vi "Example.vi"() -> ()   [LabVIEW 2014, in "Nephelometer.lvclass"]
uses:
  Nephelometer.lvclass
  Reusable/Session APIs/File Access/Config Data/Config Session.ctl
  Reusable/Session APIs/File Access/Config Data/Config Data.lvclass
  Configurable Device/Configurable Device.lvclass/Configurable Device.ctl
  Reusable/Session APIs/Serial/Serial Session.lvclass
  Nephelometer.lvclass/Nephelometer.ctl
  Configurable Device/Write Handle.vi
  <userlib>/_Session Fwk/Session - Root.lvclass
panel:
  out "error out 6":errorcluster
  in  "Fan Power":bool
  in  "Lamp Power":bool
  in  "position":enum16{"Total", "Back"}(ring)
  in  "Power":bool=TRUE
  out "Aux Data":T1
  out "Data Record":T2
  in  "Zero":bool
  out "Autozero Mode":i32
  out "error out 5":errorcluster
  out "current time":timestamp
  out "error out 4":errorcluster
  out "error out 3":errorcluster
  in  "Valve":bool
  in  "Blower":u8(slide) scale=0.0..255.0
  out "error out":errorcluster
  out "Vlamp":cluster{"Voltage":dbl, "Amperage":dbl}
  out "Tsample":dbl
  out "Tinlet":dbl
  out "RH":dbl
  out "Pressure":dbl
  out "error out 2":errorcluster
  out "RD":string
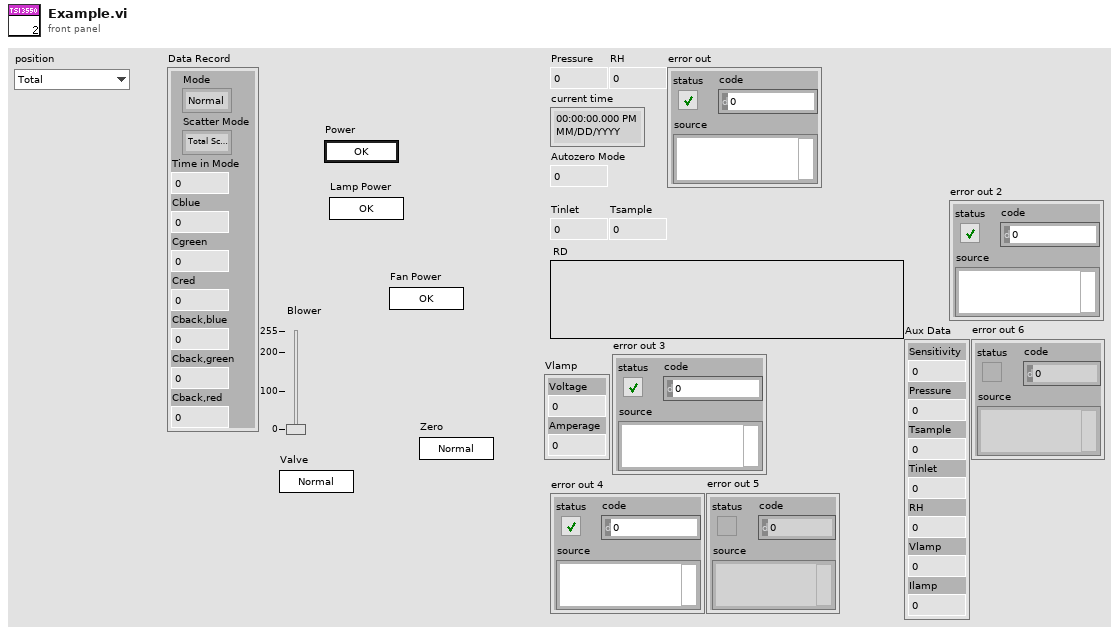
[diagram p1: front panel]
types:
  T1 = cluster{"Sensitivity":dbl, "Pressure":dbl, "Tsample":dbl, "Tinlet":dbl, "RH":dbl, "Vlamp":dbl, "Ilamp":dbl}
  T2 = cluster{"Mode":enum16{"Normal", "Zero", "Blank"}, "Scatter Mode":enum16{"Total Scatter", "Back Scatter"}, "Time in Mode":dbl, "Cblue":i32, "Cgreen":dbl, "Cred":dbl, "Cback,blue":dbl, "Cback,green":dbl, "Cback,red":dbl}
  T3 = typedef "Config Data.lvclass/Config Session.ctl" = refnum<data-value>
  T4 = typedef "Session - Root.lvclass/Session Handle.ctl" = refnum<data-value>
  T5 = cluster{"Mode":enum16{"Normal", "Zero", "Blank"}, "Scatter Mode":enum16{"Total Scatter", "Back Scatter"}, "Time in Mode":i32, "Cblue":dbl, "Cgreen":dbl, "Cred":dbl, "Cback,blue":dbl, "Cback,green":dbl, "Cback,red":dbl}
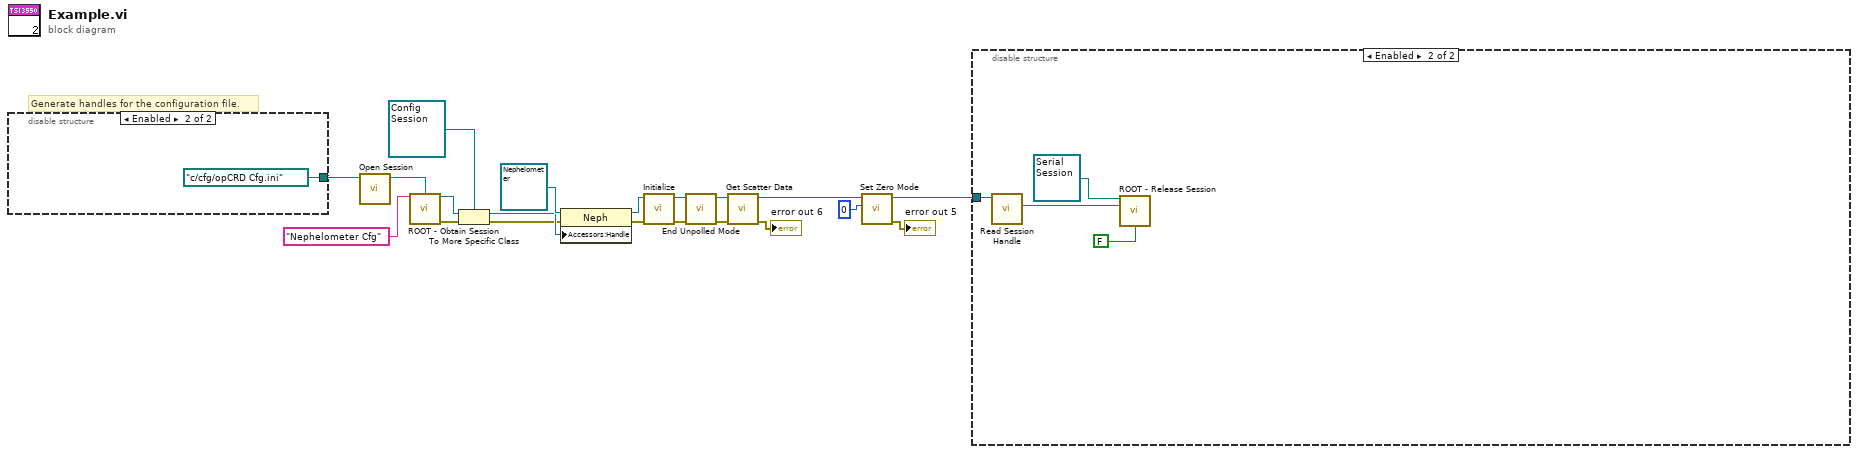
[diagram p0: block diagram]
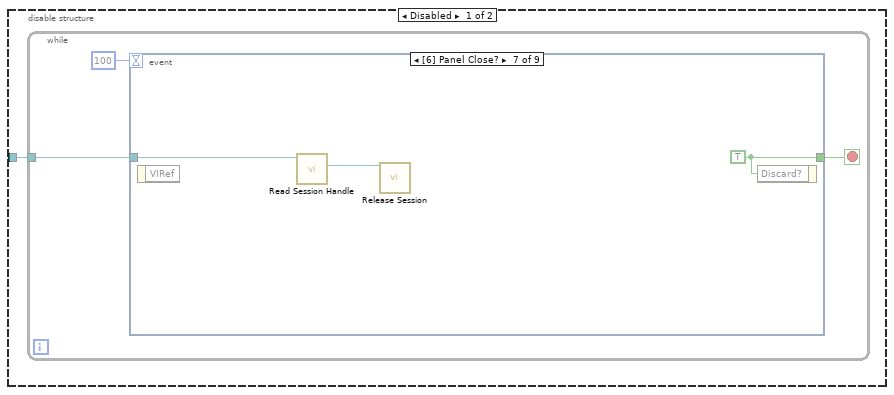
[diagram p2: hidden frame]
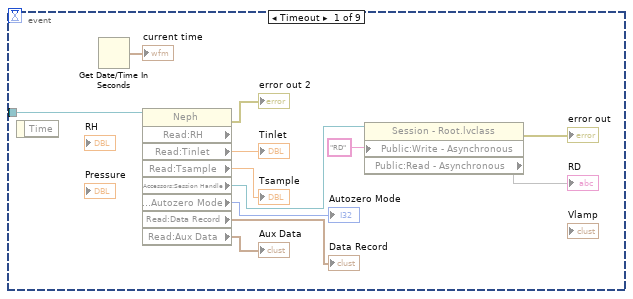
[diagram p3: hidden frame]
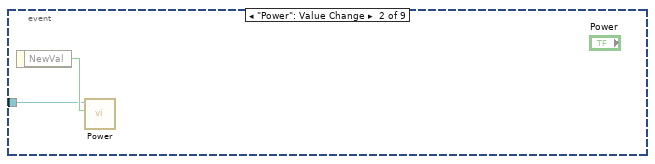
[diagram p4: hidden frame]
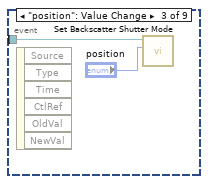
[diagram p5: hidden frame]
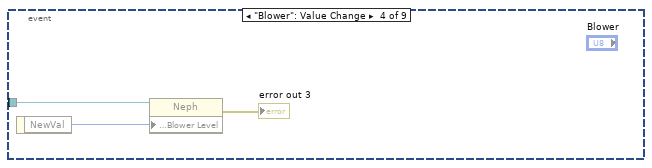
[diagram p6: hidden frame]
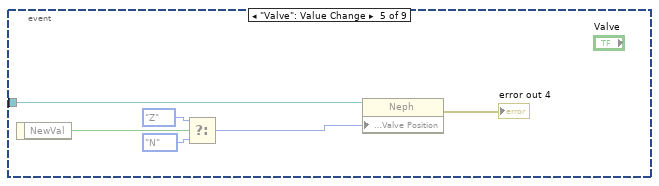
[diagram p7: hidden frame]
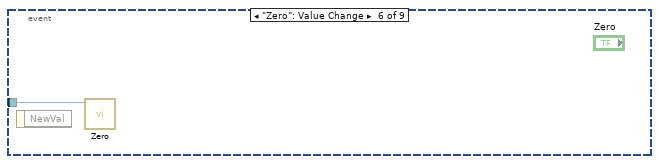
[diagram p8: hidden frame]
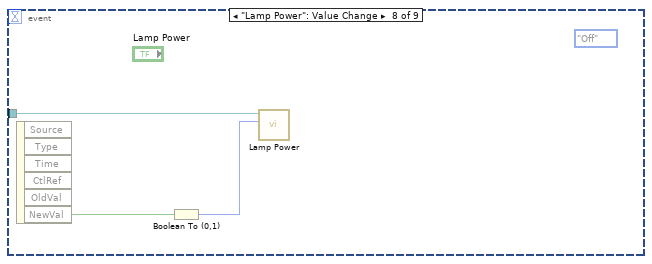
[diagram p9: hidden frame]
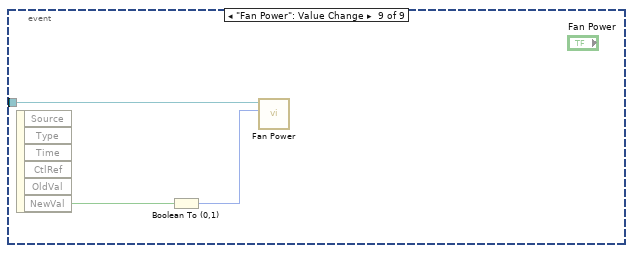
[diagram p10: hidden frame]
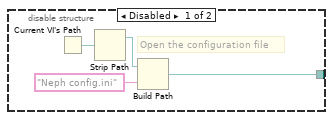
[diagram p11: hidden frame]
diagram:
  # "Generate handles for the configuration file."
  n1 = disable-structure shown="Enabled" {
    disable-tunnel: [w21 path "c:/cfg/opCRD Cfg.ini" ("Path")] -> w17
    frame Disabled {
      # "Open the configuration file"
      n2 = Current VI's Path() -> (path=w24:path)
      n3 = Strip Path(path=w24) -> (stripped path=w23:path)  [unwired: 1 out]
      n4 = Build Path(base path=w23, name or relative path="Neph config.ini") -> (appended path=w21:path)
    }
    frame Enabled {
    }
  }
  n5 = call "Open Session.vi"("Path"=w17) -> ("Config Data"=w20:refnum<class "Config Data.lvclass">)  [unwired: 9 in, 1 out]
  n6 = call <userlib>:"ROOT - Obtain Session.vi"("Session Name ()"="Nephelometer Cfg", "OBJ - Session"=w20) -> ("Session Handle"=w16:T4, "error out"=w15:errorcluster)  [unwired: 11 in, 1 out]
  n7 = To More Specific Class(target class=T3 refnum ("Session Handle"), reference=w16, error in=w15) -> (specific class reference=w13:T3, error out=w12:errorcluster)
  n8 = property class="Neph"(reference=refnum<class "Nephelometer.lvclass"> refnum ("Neph"), error in=w12, "Accessors:Handle"=w13) -> (reference out=w11:refnum<class "Nephelometer.lvclass">, error out=w10:errorcluster)
  n9 = call "Initialize.vi"("error in"=w10, "Neph In"=w11) -> ("error out"=w8:errorcluster, "Neph Out"=w9:refnum<class "Nephelometer.lvclass">)  [unwired: 8 in]
  n10 = call "End Unpolled Mode.vi"("error in"=w8, "Neph in"=w9) -> ("error out"=w3:errorcluster, "Neph out"=w4:refnum<class "Nephelometer.lvclass">)  [unwired: 8 in]
  n11 = call "Get Scatter Data.vi"("error in"=w3, "Neph in"=w4) -> ("error out"=→"error out 6":errorcluster, "Neph out"=w2:refnum<class "Nephelometer.lvclass">)  [unwired: 7 in, 1 out]
  n12 = call "Set Zero Mode.vi"("Mode"=u8 0, "Neph in"=w2) -> ("error out"=→"error out 5":errorcluster, "Neph out"=w7:refnum<class "Nephelometer.lvclass">)  [unwired: 8 in]
  n13 = disable-structure shown="Enabled" {
    disable-tunnel: w7 -> [w26 w68]
    frame Disabled {
      n14 = while {
        tunnel: w26 -> [w27]
        stop <- w29 stop-if-true
        n15 = event shown="[6] Panel Close?" {
          selector: _ -> [_ _ _ _ _ _ _ _ _]
          dyn-events: _ -> [_ _ _ _ _ _ _ _ _]
          timeout: 100 -> [_ _ _ _ _ _ _ _ _]
          tunnel: [_ _ _ _ _ _ w58 _ _] -> w29
          tunnel: w27 -> [w36 w42 w45 w48 w54 w55 w56 w61 w63]
          event Timeout {
            n16 = event-data() -> ()  [unwired: 1 in, 1 out]
            n17 = Get Date/Time In Seconds() -> (seconds since 1Jan1904=→"current time":timestamp)
            n18 = property class="Neph" props=["Read:RH", "Read:Tinlet", "Read:Tsample", "Accessors:Session Handle", "Commands:Autozero Mode", "Read:Data Record", "Read:Aux Data"](reference=w36) -> (error out=→"error out 2":errorcluster, "Read:Tinlet"=→"Tinlet":dbl, "Read:Tsample"=→"Tsample":dbl, "Accessors:Session Handle"=w35:T4, "Commands:Autozero Mode"=→"Autozero Mode":u8, "Read:Data Record"=→"Data Record":T5, "Read:Aux Data"=→"Aux Data":T1)  [unwired: 1 in, 2 out]
            n19 = property class="Session - Root.lvclass"(reference=w35, "Public:Write - Asynchronous"="RD" ("Write - Asynchronous")) -> (error out=→"error out":errorcluster, "Public:Read - Asynchronous"=→"RD")  [unwired: 1 in, 1 out]
          }
          event "Power": Value Change {
            n20 = event-data() -> ("NewVal"=w43:bool)  [unwired: 1 in]
            n21 = call "Power.vi"("Power?"=w43, "Neph in"=w42) -> ()  [unwired: 8 in, 2 out]
          }
          event "position": Value Change {
            n22 = event-data() -> ()  [unwired: 1 in, 6 out]
            n23 = call "Set Backscatter Shutter Mode.vi"("position"="position", "Neph in"=w45) -> ()  [unwired: 8 in, 2 out]
          }
          event "Blower": Value Change {
            n24 = event-data() -> ("NewVal"=w47:u8)  [unwired: 1 in]
            n25 = property class="Neph"(reference=w48, "Commands:Blower Level"=w47) -> (error out=→"error out 3":errorcluster)  [unwired: 1 in, 1 out]
          }
          event "Valve": Value Change {
            n26 = event-data() -> ("NewVal"=w53:bool)  [unwired: 1 in]
            n27 = Select(t=enum16{"N", "Z"}."Z" ("Valve Position"), s=w53, f=enum16{"N", "Z"}."N" ("Valve Position")) -> (s? t:f=w50:enum16{"N", "Z"})
            n28 = property class="Neph"(reference=w54, "Commands:Valve Position"=w50) -> (error out=→"error out 4":errorcluster)  [unwired: 1 in, 1 out]
          }
          event "Zero": Value Change {
            n29 = event-data() -> ()  [unwired: 1 in, 1 out]
            n30 = call "Zero.vi"("Neph in"=w55) -> ()  [unwired: 9 in, 2 out]
          }
          event Panel Close? {
            w58 = TRUE ("Discard?")
            n31 = event-data() -> ()  [unwired: 1 in, 1 out]
            n32 = call "Read Session Handle.vi"("Nephelometer in"=w56) -> ("Session Handle"=w57:T4)  [unwired: 8 in, 2 out]
            n33 = call "Release Session.vi"("Session Handle"=w57) -> ()  [unwired: 14 in, 1 out]
            n34 = event-data("Discard?"=w58) -> ()  [unwired: 1 in, 1 out]
          }
          event "Lamp Power": Value Change {
            (unwired) enum16{"Off", "On"}."Off" ("On/Off")
            n35 = event-data() -> ("NewVal"=w60:bool)  [unwired: 1 in, 5 out]
            n36 = Boolean To (0,1)(Boolean=w60) -> (0, 1=w59:i16)
            n37 = call "Lamp Power.vi"("On/Off"=w59, "Neph in"=w61) -> ()  [unwired: 8 in, 2 out]
          }
          event "Fan Power": Value Change {
            n38 = event-data() -> ("NewVal"=w64:bool)  [unwired: 1 in, 5 out]
            n39 = Boolean To (0,1)(Boolean=w64) -> (0, 1=w62:i16)
            n40 = call "Fan Power.vi"("On/Off"=w62, "Neph in"=w63) -> ()  [unwired: 8 in, 2 out]
          }
        }
      }
    }
    frame Enabled {
      n41 = call "Read Session Handle.vi"("Nephelometer in"=w68) -> ("Session Handle"=w67:T4)  [unwired: 8 in, 2 out]
      n42 = call <userlib>:"ROOT - Release Session.vi"("OBJ - Session in"=refnum<class "Serial Session.lvclass"> refnum ("Serial Session"), "Session Handle in"=w67, "force destroy? (F)"=FALSE) -> ()  [unwired: 11 in, 2 out]
    }
  }
